vi "Created Queues.vi"(6 "Created Queue Alias":string, 7 "jettl in":refnum<class "jettl.lvclass">, 8 "Priority?":bool, 9 "Msg Strategy":refnum<class "Msg Strategy.lvclass">, 10 "Queue Mailbox":refnum<data-value>) -> (5 "jettl out":refnum<class "jettl.lvclass">)   [LabVIEW 2021, in "jettl.lvlib" / "Queue Mailbox.lvlib"]
uses:
  Queue Mailbox.lvlib
  Self Queue/Self Queue.lvlib
  jettl.lvlib
  jettl/jettl.lvclass
  Msg Strategy/Msg Strategy.lvclass
  Queue Mailbox/Queue Mailbox.lvclass
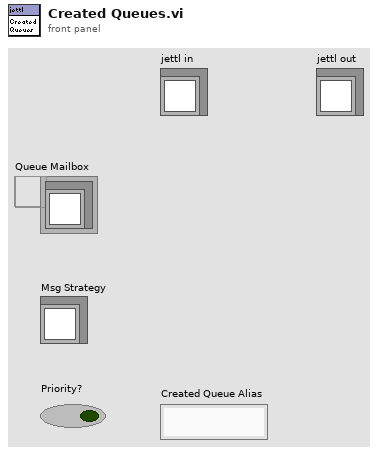
[diagram p1: front panel]
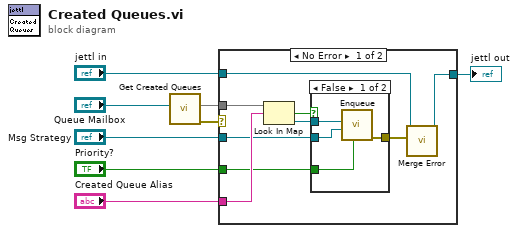
[diagram p0: block diagram]
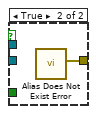
[diagram p2: hidden frame]
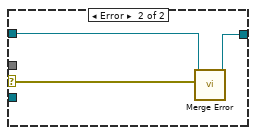
[diagram p3: hidden frame]
diagram:
  n1 = call "Get Created Queues.vi"("Queue Mailbox"="Queue Mailbox") -> ("error out"=w1:errorcluster, "Created Queues"=w3:map{string, refnum<data-value>})  [unwired: 9 in]
  n2 = case shown="No Error" w1 {
    selector: w1 -> [_ w23]
    tunnel: "Created Queue Alias" -> [w14 _]
    tunnel: "Priority?" -> [w13 _]
    tunnel: "Msg Strategy" -> [w12 _]
    tunnel: [w11 w24] -> w5
    tunnel: "jettl in" -> [w10 w25]
    tunnel: w3 -> [w9 _]
    frame No Error {
      n3 = Look In Map(map=w9, key=w14) -> (key not found?=w16:bool, value=w17:refnum<data-value>)  [unwired: 1 in]
      n4 = case shown="False" w16 {
        tunnel: [w21 w22] -> w15
        tunnel: w13 -> [w20 _]
        tunnel: w12 -> [w19 _]
        tunnel: w17 -> [w18 _]
        frame False {
          n5 = call "Enqueue.vi"("Priority?"=w20, "Msg Strategy"=w19, "Self Queue"=w18) -> ("error out"=w21:errorcluster)  [unwired: 8 in]
        }
        frame True {
          n6 = call "Alias Does Not Exist Error.vi"() -> ("Error"=w22:errorcluster)  [unwired: 11 in]
        }
      }
      n7 = call-dynamic "Merge Error.vi"("Error"=w15, "Merge Error in"=w10) -> ("Merge Error out"=w11:refnum<class "jettl.lvclass">)  [unwired: 9 in]
    }
    frame Error {
      n8 = call-dynamic "Merge Error.vi"("Error"=w23, "Merge Error in"=w25) -> ("Merge Error out"=w24:refnum<class "jettl.lvclass">)  [unwired: 9 in]
    }
  }
  "jettl out" <- w5
